vi "CVT_DATA.vi"(7 "경로":path, 8 "error in":errorcluster caption="error IN", 9 "DATA":sgl[][](array[numeric]), 10 "10_Count_In":u32, 11 "ref_file_in":refnum<file>) -> (0 "error out":errorcluster, 2 "10_Count_Out":u32, 3 "ref_file_Out":refnum<file>)   [LabVIEW 2023]
panel:
  in  "숫자형":u32
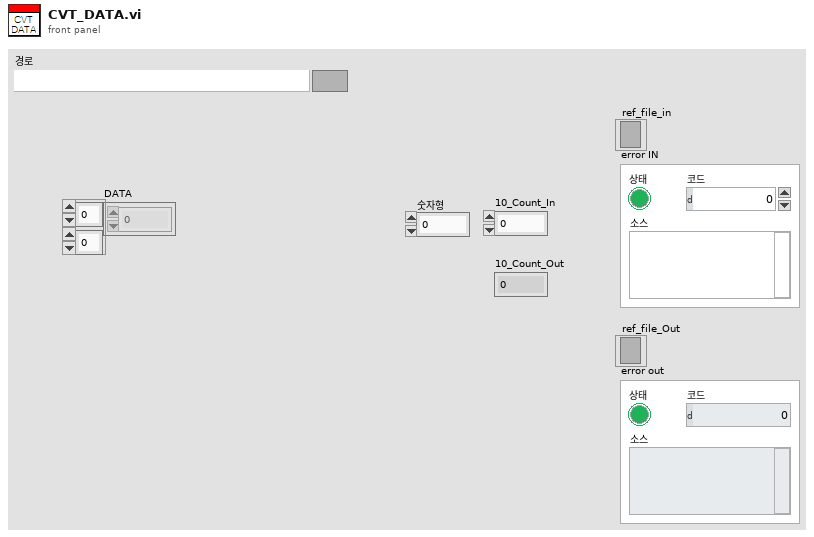
[diagram p1: front panel]
types:
  T1 = enum16{"open", "replace", "create", "open or create", "replace or create", "replace or create with confirmation"}
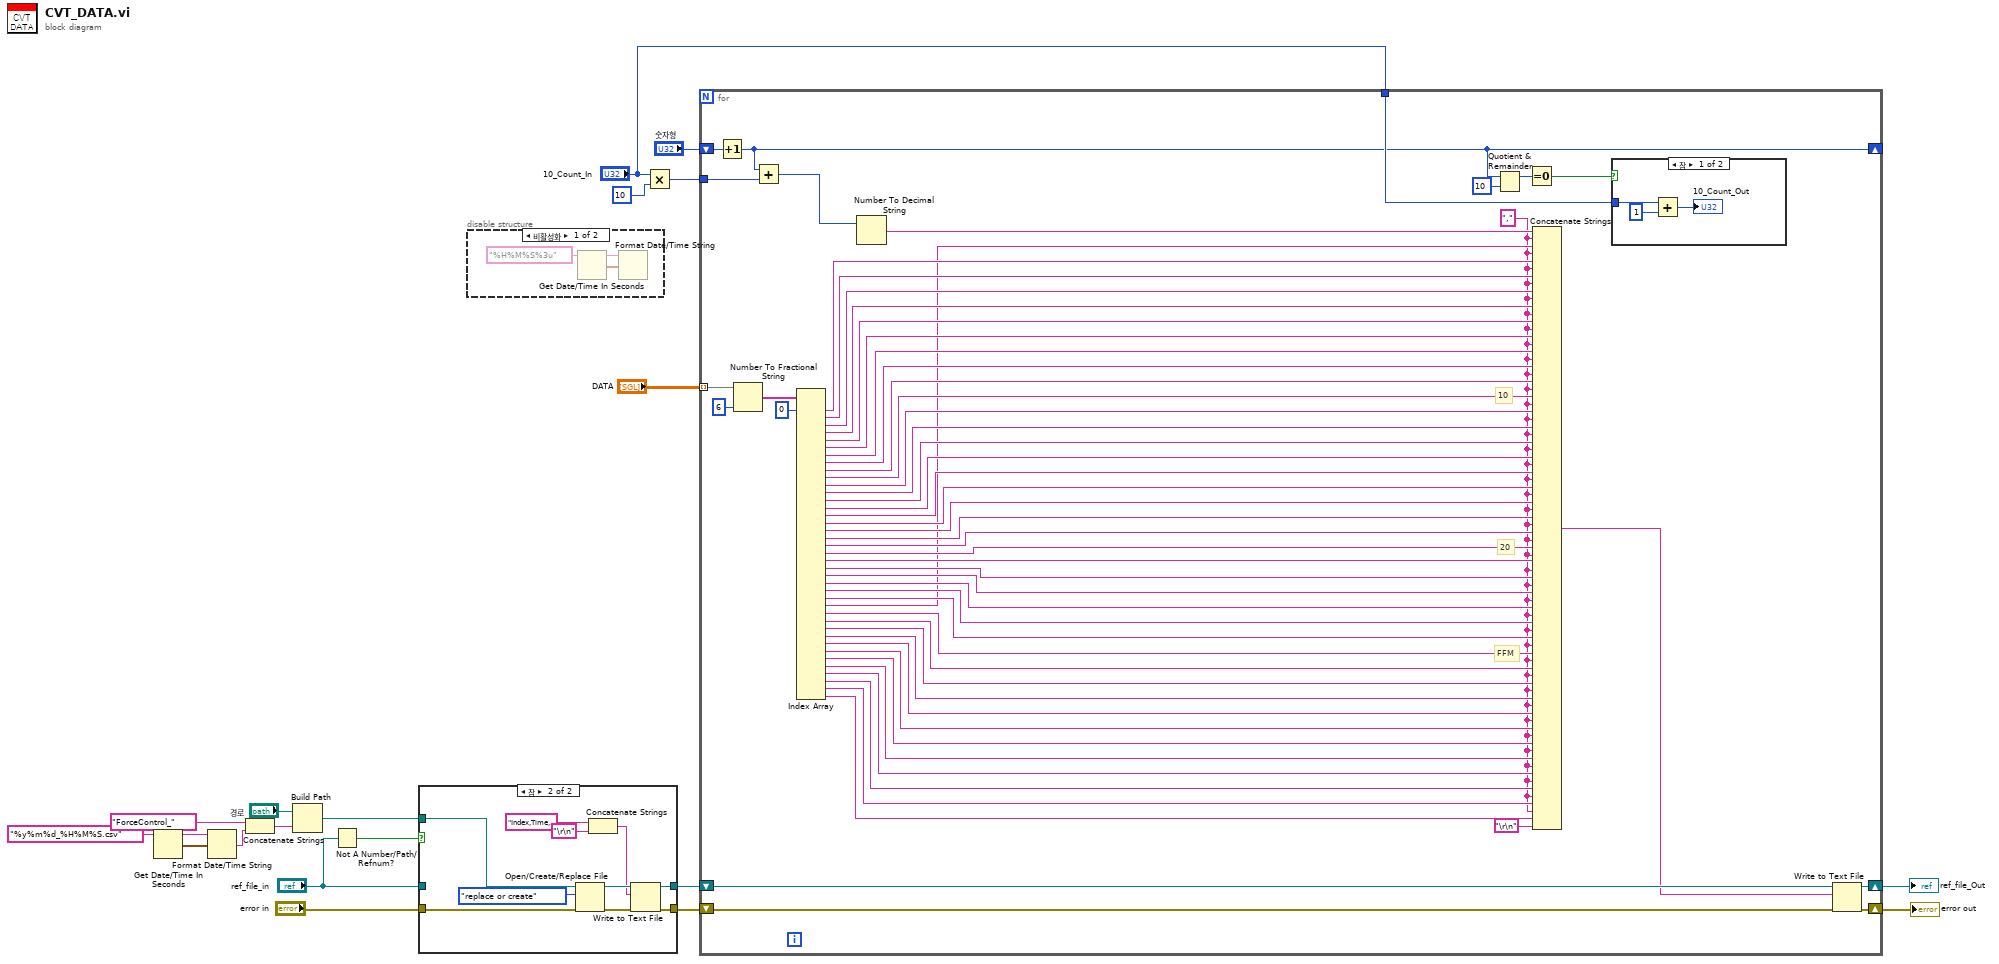
[diagram p0: block diagram]
diagram:
  n1 = Get Date/Time In Seconds() -> (seconds since 1Jan1904=w12:timestamp)
  n2 = Format Date/Time String(time format string (%c)="%y%m%d_%H%M%S.csv" ("시간 포맷 문자열 (%c)"), seconds (now)=w12) -> (date/time string=w6:string)  [unwired: 1 in]
  n3 = Concatenate Strings("ForceControl_" ("문자열"), w6) -> (w7:string)
  n4 = Build Path(base path="경로", name or relative path=w7) -> (appended path=w9:path)
  n5 = Not A Number/Path/Refnum?(number/path/refnum="ref_file_in") -> (NaN/Path/Refnum?=w17:bool)
  n6 = case shown="참" w17 {
    tunnel: "ref_file_in" -> [w21 _]
    tunnel: [w21 w27] -> w15
    tunnel: [w20 w26] -> w14
    tunnel: "error in" -> [w20 w28]
    tunnel: w9 -> [_ w25]
    frame False {
    }
    frame True {
      n7 = Open/Create/Replace File(file path (use dialog)=w25, error in=w28, operation (0:open)=T1."replace or create" ("동작(0:open)")) -> (refnum out=w31:refnum<file>, error out=w30:errorcluster)  [unwired: 3 in, 1 out]
      n8 = Concatenate Strings("Index,Time,L_Roll,L_AngVel,L_Force,R_Roll,Belly_accZ,R_AngVel,R_Force,L_Ref_Force,R_Ref_Force,L_D_Current,R_D_Current,L_A_Current,R_A_Current,L_D_Vel,R_D_Vel,L_A_Vel,R_A_Vel,L_D_Pos,R_D_Pos,L_A_Pos,R_A_Pos,L_GCP,R_GCP,L_ForceMode,R_ForceMode,OptimizeDone,L_Error_Pull,L_C1_Pull,L_C2_Pull,R_Error_Pull,R_C1_Pull,R_C2_Pull,L_Error_Release,L_C1_Release,L_C2_Release,R_Error_Release,R_C1_Release,R_C2_Release" ("텍스트"), "\r\n") -> (w23:string)
      n9 = Write to Text File(file (use dialog)=w31, text=w23, error in=w30) -> (refnum out=w27:refnum<file>, error out=w26:errorcluster)  [unwired: 1 in, 1 out]
    }
  }
  n10 = disable-structure shown="비활성화" {
    frame Disabled {
      n11 = Get Date/Time In Seconds() -> (seconds since 1Jan1904=w33:timestamp)
      n12 = Format Date/Time String(time format string (%c)="%H%M%S%3u" ("시간 포맷 문자열 (%c)"), seconds (now)=w33) -> ()  [unwired: 1 in, 1 out]
    }
    frame Enabled {
    }
  }
  n13 = Multiply(x="10_Count_In", y=u32 10) -> (x*y=w3:u32)
  n14 = for {
    tunnel: "DATA" -> [w52] mode=indexing
    shift-right: [w92] -> w19
    shift-left: w15 -> [w91]
    shift-right: [w90] -> w18
    shift-left: w14 -> [w89]
    shift-right: [w85] -> _
    shift-left: "숫자형" -> [w86]
    tunnel: w3 -> [w88]
    tunnel: "10_Count_In" -> [w87]
    w35 = "," ("문자열")
    # "FFM"
    # "20"
    # "10"
    n15 = Increment(x=w86) -> (x+1=w85:u32)
    n16 = Number To Fractional String(number=w52, precision (6)=i16 6 ("정밀도(6)")) -> (F-format string=w79:string[])  [unwired: 2 in]
    n17 = Add(x=w85, y=w88) -> (x+y=w51:u32)
    n18 = Index Array(array=w79, index #1=0 ("인덱스")) -> (element #1=w77:string, element #2=w76:string, element #3=w75:string, element #4=w74:string, element #5=w73:string, element #6=w72:string, element #7=w71:string, element #8=w70:string, element #9=w69:string, element #10=w68:string, element #11=w67:string, element #12=w66:string, element #13=w65:string, element #14=w64:string, element #15=w63:string, element #16=w62:string, element #17=w61:string, element #18=w60:string, element #19=w59:string, element #20=w58:string, element #21=w57:string, element #22=w56:string, element #23=w55:string, element #24=w54:string, element #25=w53:string, element #26=w49:string, element #27=w48:string, element #28=w42:string, element #29=w47:string, element #30=w46:string, element #31=w45:string, element #32=w44:string, element #33=w43:string, element #34=w41:string, element #35=w40:string, element #36=w39:string, element #37=w38:string, element #38=w37:string, element #39=w36:string)  [unwired: 38 in]
    n19 = Number To Decimal String(number=w51) -> (decimal integer string=w78:string)  [unwired: 1 in]
    n20 = Quotient & Remainder(x=w85, y=u32 10) -> (x-y*floor(x/y)=w83:u32)  [unwired: 1 out]
    n21 = Equal To 0?(x=w83) -> (x = 0?=w82:bool)
    n22 = Concatenate Strings(w78, w35, w48, w35, w77, w35, w76, w35, w75, w35, w74, w35, w73, w35, w72, w35, w71, w35, w70, w35, w69, w35, w68, w35, w67, w35, w66, w35, w65, w35, w64, w35, w63, w35, w62, w35, w61, w35, w60, w35, w59, w35, w58, w35, w57, w35, w56, w35, w55, w35, w54, w35, w53, w35, w49, w35, w42, w35, w47, w35, w46, w35, w45, w35, w44, w35, w43, w35, w41, w35, w40, w35, w39, w35, w38, w35, w37, w35, w36, "\r\n") -> (w50:string)
    n23 = case shown="참" w82 {
      tunnel: w87 -> [w95 _]
      frame True {
        n24 = Add(x=w95, y=u32 1) -> (x+y=→"10_Count_Out":u32)
      }
      frame False {
      }
    }
    n25 = Write to Text File(file (use dialog)=w91, text=w50, error in=w89) -> (refnum out=w92:refnum<file>, error out=w90:errorcluster)  [unwired: 1 in, 1 out]
  }
  "ref_file_Out" <- w19
  "error out" <- w18
